vi "Maxi Gauge-convert6int.vi"(0 "Integer1 in":u8, 1 "String in":string, 2 "W/R [W: Int in; Str out ]":bool, 5 "Integer2 in":u8, 7 "Integer3 in":u8, 9 "Integer4 in":u8, 11 "Integer5 in":u8, 12 "Integer6 in":u8) -> (3 "String out":string, 4 "Integer1 out":u8, 6 "Integer2 out":u8, 8 "Integer3 out":u8, 10 "Integer4 out":u8, 14 "Integer6 out":u8, 15 "Integer5 out":u8)   [LabVIEW 2013, in "Maxi Gauge.lvlib"]
uses:
  <instrlib>/Maxi Gauge/Maxi Gauge.lvlib
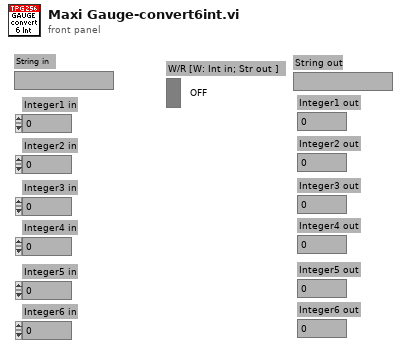
[diagram p1: front panel]
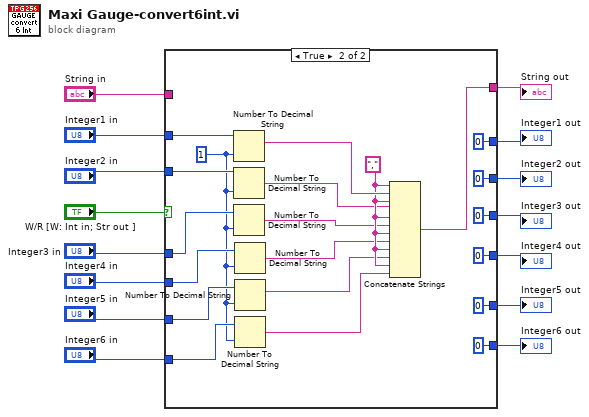
[diagram p0: block diagram]
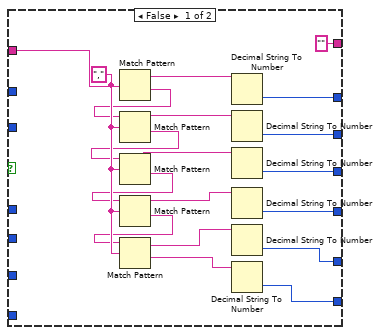
[diagram p2: hidden frame]
diagram:
  n1 = case shown="True" "W/R [W: Int in; Str out ]" {
    tunnel: "Integer1 in" -> [_ w55]
    tunnel: "Integer2 in" -> [_ w54]
    tunnel: "Integer3 in" -> [_ w53]
    tunnel: "Integer4 in" -> [_ w52]
    tunnel: "Integer5 in" -> [_ w51]
    tunnel: "Integer6 in" -> [_ w50]
    tunnel: ["" w48] -> w8
    tunnel: "String in" -> [w34 _]
    tunnel: [w22 0] -> w6
    tunnel: [w21 0] -> w5
    tunnel: [w20 0] -> w4
    tunnel: [w19 0] -> w3
    tunnel: [w18 0] -> w2
    tunnel: [w17 0] -> w1
    frame False {
      w32 = "," ("regular expression")
      n2 = Match Pattern(string=w34, regular expression=w32) -> (before substring=w33:string, after substring=w31:string)  [unwired: 1 in, 2 out]
      n3 = Match Pattern(string=w31, regular expression=w32) -> (before substring=w26:string, after substring=w30:string)  [unwired: 1 in, 2 out]
      n4 = Match Pattern(string=w30, regular expression=w32) -> (before substring=w25:string, after substring=w29:string)  [unwired: 1 in, 2 out]
      n5 = Match Pattern(string=w29, regular expression=w32) -> (before substring=w24:string, after substring=w28:string)  [unwired: 1 in, 2 out]
      n6 = Match Pattern(string=w28, regular expression=w32) -> (before substring=w23:string, after substring=w27:string)  [unwired: 1 in, 2 out]
      n7 = Decimal String To Number(string=w33) -> (number=w22:i32)  [unwired: 2 in, 1 out]
      n8 = Decimal String To Number(string=w26) -> (number=w21:i32)  [unwired: 2 in, 1 out]
      n9 = Decimal String To Number(string=w25) -> (number=w20:i32)  [unwired: 2 in, 1 out]
      n10 = Decimal String To Number(string=w24) -> (number=w19:i32)  [unwired: 2 in, 1 out]
      n11 = Decimal String To Number(string=w23) -> (number=w18:i32)  [unwired: 2 in, 1 out]
      n12 = Decimal String To Number(string=w27) -> (number=w17:i32)  [unwired: 2 in, 1 out]
    }
    frame True {
      w40 = ","
      w49 = i16 1 ("width (-)")
      n13 = Number To Decimal String(number=w55, width (-)=w49) -> (decimal integer string=w41:string)
      n14 = Number To Decimal String(number=w54, width (-)=w49) -> (decimal integer string=w39:string)
      n15 = Number To Decimal String(number=w53, width (-)=w49) -> (decimal integer string=w38:string)
      n16 = Number To Decimal String(number=w52, width (-)=w49) -> (decimal integer string=w37:string)
      n17 = Number To Decimal String(number=w51, width (-)=w49) -> (decimal integer string=w36:string)
      n18 = Number To Decimal String(number=w50, width (-)=w49) -> (decimal integer string=w35:string)
      n19 = Concatenate Strings(w40, w41, w40, w39, w40, w38, w40, w37, w40, w36, w40, w35) -> (w48:string)
    }
  }
  "Integer1 out" <- w6
  "Integer2 out" <- w5
  "Integer3 out" <- w4
  "Integer4 out" <- w3
  "Integer5 out" <- w2
  "Integer6 out" <- w1
  "String out" <- w8
